vi "Read Value.vi"(8 "error in (no error)":errorcluster, 11 "Column in":refnum<class "Column.lvclass">) -> (0 "error out":errorcluster, 2 "Value":string, 3 "Column out":refnum<class "Column.lvclass">)   [LabVIEW 2020]
uses:
  Column.lvclass
  C:/Users/User/Desktop/Raman Program/Database OOP/source/Database OOP/Column/Column Class/Column.lvclass
  C:/Users/User/Desktop/Raman Program/Database OOP/source/Database OOP/Column Interface/Column Interface.lvclass
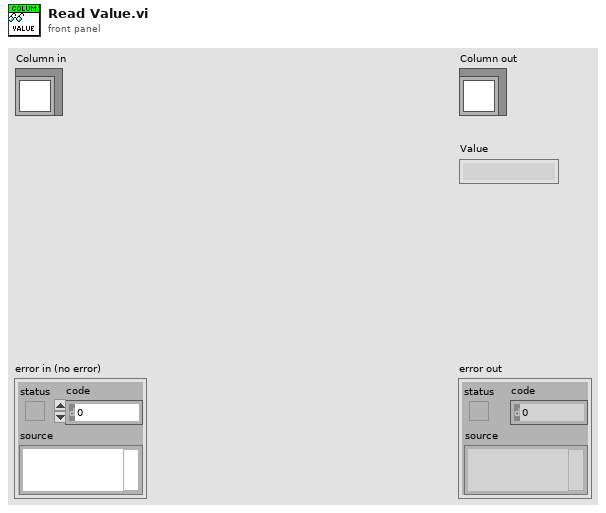
[diagram p1: front panel]
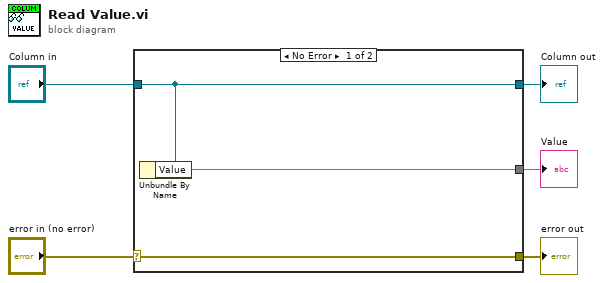
[diagram p0: block diagram]
diagram:
  n1 = case shown="No Error" "error in (no error)" {
    selector: "error in (no error)" -> [w8 w9]
    tunnel: [w8 w9] -> w4
    tunnel: [w7 w10] -> w2
    tunnel: "Column in" -> [w7 w10]
    tunnel: [w6 _] -> w1
    frame No Error {
      n2 = Unbundle By Name(w7) -> ("Value"=w6)
    }
    frame Error {
    }
  }
  "error out" <- w4
  "Column out" <- w2
  "Value" <- w1
